vi "Front Panel Layout.vi"(4 "bounds (panel bounds)":T1, 6 "defer panel updates (F)":bool, 7 "scaling settings":T2={"scaling type"=enum."Scale layout to fit panel", "scale text"=TRUE}, 8 "error in (no error)":errorcluster, 10 "panel layout file":path, 11 "VI refnum":refnum<vi>) -> (0 "error out":errorcluster)   [LabVIEW 2015]
uses:
  <vilib>/Front Panel Layout/Scaling Settings.ctl
  <vilib>/Front Panel Layout/Scaling Type.ctl
  <vilib>/Front Panel Layout/Bounds Type.ctl
  <vilib>/Front Panel Layout/VI Panel Layout/VI Panel Layout.lvclass
  <vilib>/Front Panel Layout/NI_SE_Front Panel Layout.lvlib
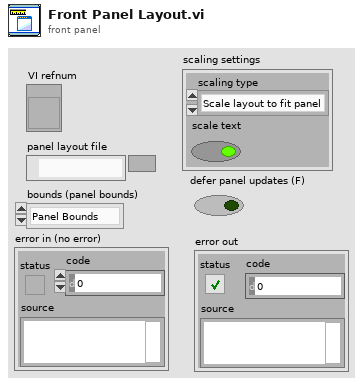
[diagram p1: front panel]
types:
  T1 = typedef "NI_SE_Front Panel Layout.lvlib/Bounds Type.ctl" = enum16{"Panel Bounds", "Window Bounds"}
  T2 = typedef "NI_SE_Front Panel Layout.lvlib/Scaling Settings.ctl" = cluster{"scaling type":T3, "scale text":bool}
  T3 = typedef "NI_SE_Front Panel Layout.lvlib/Scaling Type.ctl" = enum16{"None", "Scale panel to fit layout", "Scale layout to fit panel"}
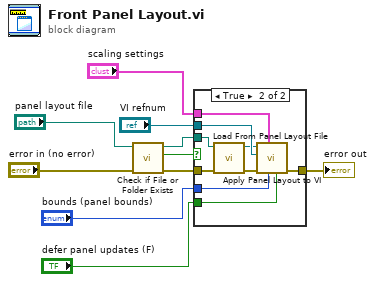
[diagram p0: block diagram]
diagram:
  n1 = call <vilib>:"Check if File or Folder Exists.vi"("error in (no error)"="error in (no error)", "path"="panel layout file") -> ("error out"=w6:errorcluster, "file or folder exists?"=w9:bool, "dup path"=w7:path)  [unwired: 7 in]
  n2 = case shown="True" w9 {
    tunnel: w6 -> [w11 w14]
    tunnel: w7 -> [_ w16]
    tunnel: "VI refnum" -> [_ w20]
    tunnel: [w11 w19] -> w1
    tunnel: "scaling settings" -> [_ w18]
    tunnel: "bounds (panel bounds)" -> [_ w13]
    tunnel: "defer panel updates (F)" -> [_ w12]
    frame False {
    }
    frame True {
      n3 = call <vilib>:"Load From Panel Layout File.vi"("error in"=w14, "panel layout file"=w16) -> ("error out"=w15:errorcluster, "panel layout out"=w17:refnum<class "VI Panel Layout.lvclass">)  [unwired: 8 in]
      n4 = call <vilib>:"Apply Panel Layout to VI.vi"("defer panel updates (F)"=w12, "bounds (panel bounds)"=w13, "scaling settings"=w18, "error in"=w15, "VI refnum"=w20, "panel layout in"=w17) -> ("error out"=w19:errorcluster)  [unwired: 4 in, 1 out]
    }
  }
  "error out" <- w1
